vi "M14_Magazine_Hardware_Implementation.vi"   [LabVIEW 2019]
uses:
  New_Magazine_Globals.vi
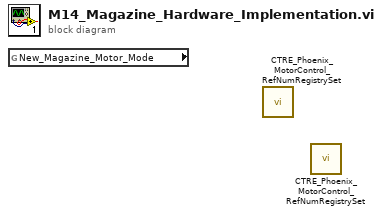
[diagram p0: block diagram]
diagram:
  n1 = global read "New_Magazine_Globals.vi" "New_Magazine_Motor_Mode"() -> ()  [unwired: 1 out]
  n2 = call <vilib>:"CTRE_Phoenix_MotorControl_RefNumRegistrySet.vi"() -> ()  [unwired: 10 in, 2 out]
  n3 = call <vilib>:"CTRE_Phoenix_MotorControl_RefNumRegistrySet.vi"() -> ()  [unwired: 10 in, 2 out]
